vi "WSVCAP SHL Host LL I2C Write.vi"(0 "C1 Data Out [DUT Ordered]":u8[][](array[numeric]) format="%.0x", 1 "Wait Ticks":u32, 2 "Slave Address":u8, 3 "Socket Mask [U64]":u64=1 format="%06x", 11 "error in":errorcluster, 12 "Sub Address":u8=20, 13 "UUT Set (0/1)":u8, 14 "FPGA":T1) -> (10 "Status":u8[](array[numeric]), 15 "error out":errorcluster)   [LabVIEW 2017]
uses:
  Type Defs/WSVCAP SHL FPGA Enum.ctl
  Type Defs/WSVCAP SHL Top Level Write Read State Enum.ctl
  Type Defs/WSVCAP SHL Transaction Enum.ctl
  Type Defs/WSVCAP SHL Top Level Control Enum.ctl
  Type Defs/WSVCAP SHL State.ctl
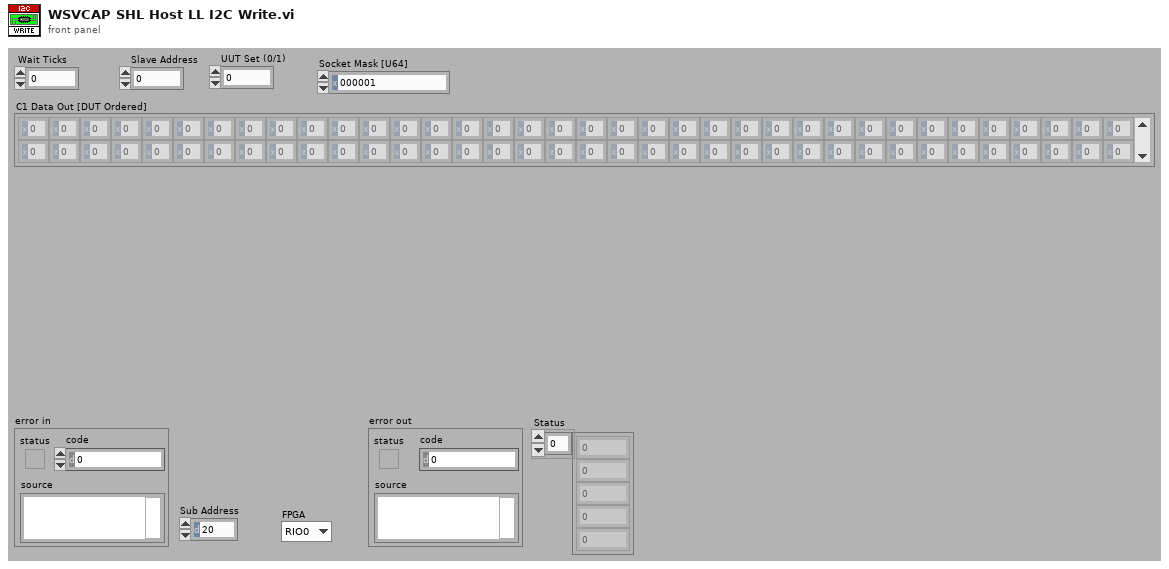
[diagram p1: front panel]
types:
  T1 = typedef "WSVCAP SHL FPGA Enum.ctl" = enum16{"RIO0", "RIO1"}
  T2 = typedef "WSVCAP SHL Top Level Write Read State Enum.ctl" = enum16{"Start", "Write", "Read", "Get Status", "Wait Until Done"}
  T3 = typedef "WSVCAP SHL Top Level Control Enum.ctl" = enum16{"Start", "Cmd", "Transaction", "Wait Ticks", "Socket Mask", "UUT Set", "Slave Address", "Sub Address", "Bytes to Write", "Bytes to Read", "Write Data", "Write Flag", "Read Data", "Read Flag", "Ack Read", "Read Status Flag", "Ack Read Status", "Status", "Cycle Count", "Stop Cycle", "Exit"}
  T4 = typedef "WSVCAP SHL Transaction Enum.ctl" = enum16{"I2C-Read Data", "I2C-Write Data", "RFFE-Ext Write", "RFFE-Ext Read", "SRL-Write Data"}
  T5 = typedef "WSVCAP SHL State.ctl" = enum8{"Idle", "Transfer Data"}
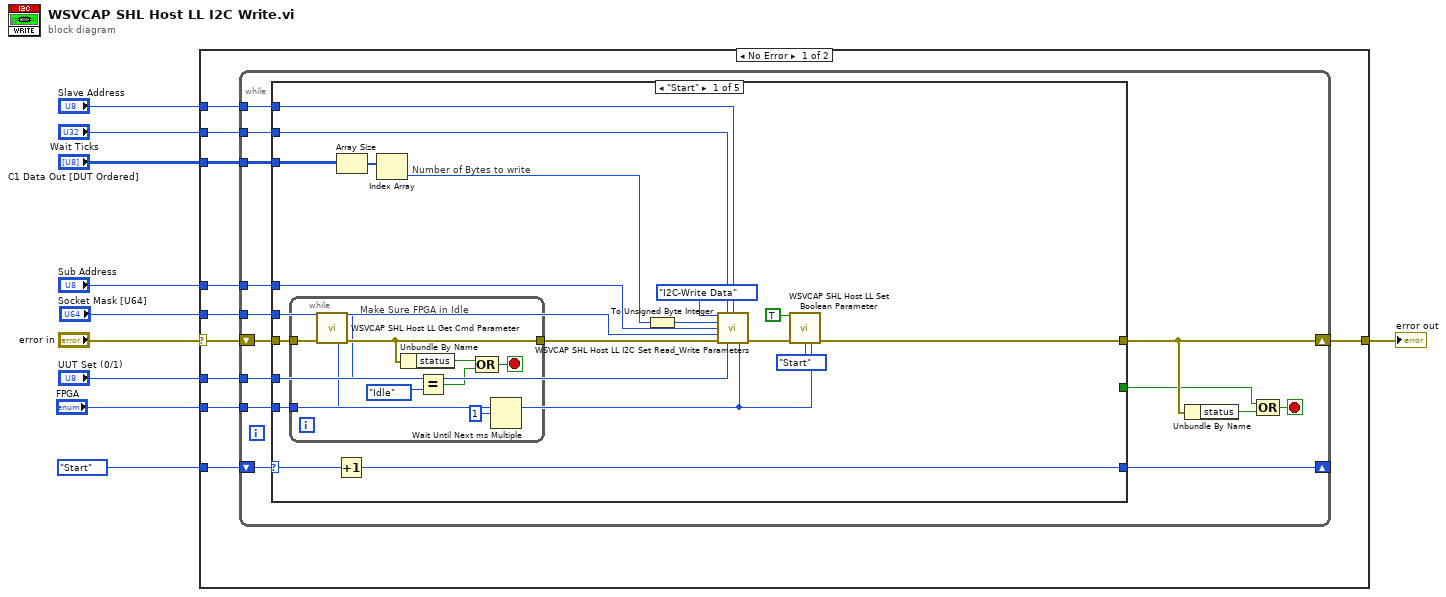
[diagram p0: block diagram]
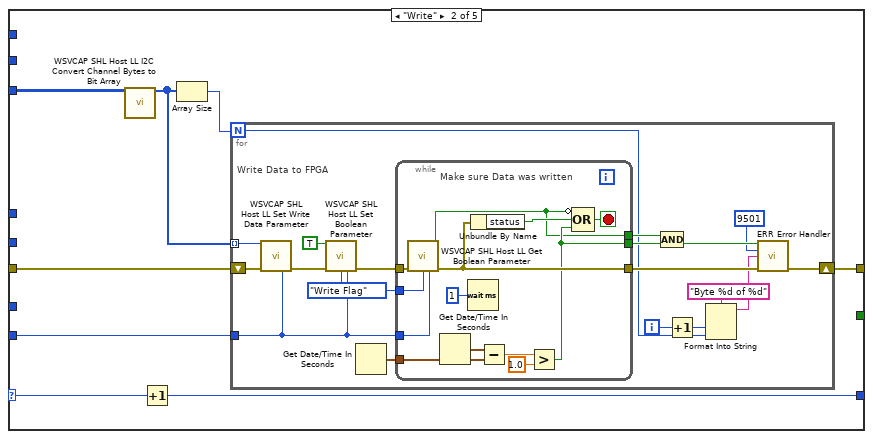
[diagram p2: hidden frame]
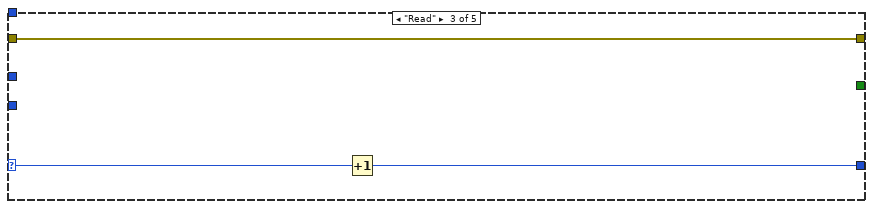
[diagram p3: hidden frame]
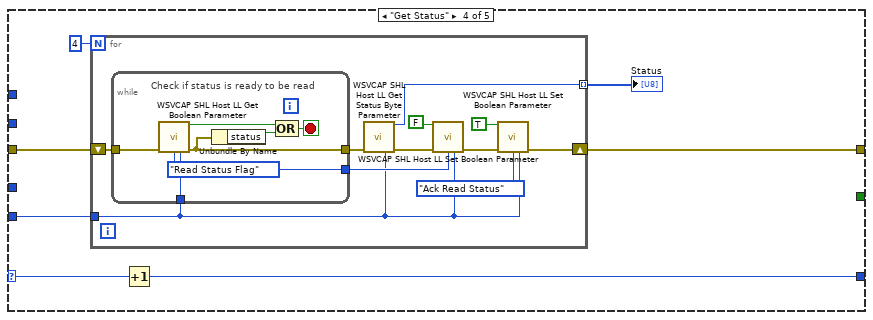
[diagram p4: hidden frame]
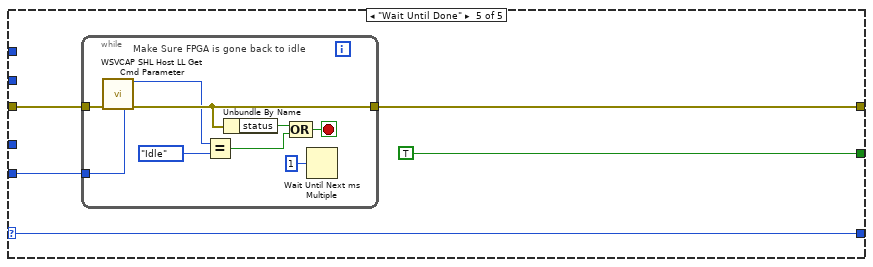
[diagram p5: hidden frame]
diagram:
  n1 = case shown="No Error" "error in" {
    selector: "error in" -> [w15 w144]
    tunnel: [w20 w144] -> w10
    tunnel: WSVCAP_SHL_Top_Level_Write_Read_State_Enum."Start" ("Write Read State") -> [w19 _]
    tunnel: "C1 Data Out [DUT Ordered]" -> [w18 _]
    tunnel: "Sub Address" -> [w17 _]
    tunnel: "Socket Mask [U64]" -> [w16 _]
    tunnel: "Wait Ticks" -> [w14 _]
    tunnel: "Slave Address" -> [w13 _]
    tunnel: "UUT Set (0/1)" -> [w12 _]
    tunnel: "FPGA" -> [w11 _]
    frame No Error {
      n2 = while {
        shift-right: [w33] -> w20
        shift-left: w15 -> [w34]
        shift-right: [w28] -> _
        shift-left: w19 -> [w29]
        tunnel: w18 -> [w27]
        tunnel: w17 -> [w26]
        tunnel: w16 -> [w25]
        tunnel: w14 -> [w24]
        tunnel: w13 -> [w23]
        tunnel: w12 -> [w22]
        tunnel: w11 -> [w21]
        stop <- w30 stop-if-true
        n3 = case shown="\"Start\"" w29 {
          selector: w29 -> [w51 w67 w103 w109 w132]
          tunnel: w34 -> [w52 w64 w104 w111 w134]
          tunnel: [w48 w69 w104 w110 w133] -> w33
          tunnel: [_ _ _ _ TRUE] -> w32
          tunnel: [w50 w68 w102 w108 w132] -> w28
          tunnel: w27 -> [w44 w63 _ _ _]
          tunnel: w26 -> [w40 _ _ _ _]
          tunnel: w25 -> [w39 _ _ _ _]
          tunnel: w24 -> [w38 _ _ _ _]
          tunnel: w23 -> [w37 _ _ _ _]
          tunnel: w22 -> [w36 _ _ _ _]
          tunnel: w21 -> [w35 w62 _ w105 w130]
          frame "Start" {
            # "Number of Bytes to write"
            n4 = while {
              tunnel: w52 -> [w57]
              tunnel: [w56] -> w49
              tunnel: w35 -> [w53]
              stop <- w61 stop-if-true
              # "Make Sure FPGA in Idle"
              n5 = call "WSVCAP SHL Host LL Get Cmd Parameter.vi"("error in (no error)"=w57, "FPGA"=w53) -> ("I2C_Cmd"=w55:T5, "error out"=w56:errorcluster)  [unwired: 12 in]
              n6 = Unbundle By Name(w56) -> ("status"=w54:bool)
              n7 = Equal?(x=w55, y=WSVCAP_SHL_State."Idle" ("Type")) -> (x = y?=w59:bool)
              n8 = Compound Arithmetic op=OR(w54, w59) -> (w61:bool)
              n9 = Wait Until Next ms Multiple(millisecond multiple=u32 1) -> ()  [unwired: 1 out]
            }
            n10 = Increment(x=w51) -> (x+1=w50:T2)
            n11 = Array Size(array=w44) -> (size(s)=w43:i32[])
            n12 = Index Array(array=w43) -> (element=w42:i32)  [unwired: 1 in]
            n13 = To Unsigned Byte Integer(number=w42) -> (unsigned 8bit integer=w41:u8)
            n14 = call "WSVCAP SHL Host LL I2C Set Read_Write Parameters.vi"("Transaction"=WSVCAP_SHL_Transaction_Enum."I2C-Write Data", "Wait Ticks"=w38, "Slave Address"=w37, "Bytes"=w41, "Sub Address [U8]"=w40, "Socket Mask [U64]"=w39, "error in (no error)"=w49, "UUT Set (0/1)"=w36, "FPGA"=w35) -> ("error out"=w48:errorcluster)  [unwired: 6 in]
            n15 = call "WSVCAP SHL Host LL Set Boolean Parameter.vi"("Boolean In"=TRUE, "error in (no error)"=w48, "FPGA Top Level Control"=WSVCAP_SHL_Top_Level_Control_Enum."Start", "FPGA"=w35) -> ()  [unwired: 11 in, 1 out]
          }
          frame "Write" {
            # "Write Data to FPGA"
            n16 = call "WSVCAP SHL Host LL I2C Convert Channel Bytes to Bit Array.vi"("C1 Data Out"=w63) -> ("Write Data"=w65:u64[])  [unwired: 14 in]
            n17 = Increment(x=w67) -> (x+1=w68:T2)
            n18 = Array Size(array=w65) -> (size(s)=w66:i32)
            n19 = for {
              N: w66 -> [w72]
              shift-right: [w80] -> w69
              shift-left: w64 -> [w88]
              tunnel: w65 -> [w87] mode=indexing
              tunnel: w62 -> [w70]
              i -> [w75]
              w83 = WSVCAP_SHL_Top_Level_Control_Enum."Write Flag" ("FPGA Top Level Control")
              n20 = call "WSVCAP SHL Host LL Set Write Data Parameter.vi"("Write Byte In"=w87, "error in (no error)"=w88, "FPGA"=w70) -> ("error out"=w86:errorcluster)  [unwired: 12 in]
              n21 = call "WSVCAP SHL Host LL Set Boolean Parameter.vi"("Boolean In"=TRUE, "error in (no error)"=w86, "FPGA Top Level Control"=w83, "FPGA"=w70) -> ("error out"=w84:errorcluster)  [unwired: 11 in]
              n22 = Get Date/Time In Seconds() -> (seconds since 1Jan1904=w82:timestamp)
              n23 = while {
                tunnel: w84 -> [w99]
                tunnel: [w98] -> w81
                tunnel: w83 -> [w97]
                tunnel: w82 -> [w94]
                tunnel: [w91] -> w79
                tunnel: [w90] -> w78
                tunnel: w70 -> [w89]
                stop <- w101 stop-if-true
                # "Make sure Data was written"
                n24 = call "WSVCAP SHL Host LL Get Boolean Parameter.vi"("error in (no error)"=w99, "FPGA Top Level Control"=w97, "FPGA"=w89) -> ("Boolean Out"=w90:bool, "error out"=w98:errorcluster)  [unwired: 11 in]
                n25 = Get Date/Time In Seconds() -> (seconds since 1Jan1904=w95:timestamp)
                n26 = Wait (ms)(milliseconds to wait=u32 1) -> ()  [unwired: 1 out]
                n27 = Unbundle By Name(w98) -> ("status"=w96:bool)
                n28 = Subtract(x=w95, y=w94) -> (x-y=w93:dbl)
                n29 = Greater?(x=w93, y=1.0) -> (0:w91:bool)
                n30 = Compound Arithmetic op=OR(invert w90, w96, w91) -> (w101:bool)
              }
              n31 = Compound Arithmetic op=AND(w78, w79) -> (w77:bool)
              n32 = Increment(x=w75) -> (x+1=w71:i32)
              n33 = Format Into String(format string="Byte %d of %d", w71, w72) -> (resulting string=w74:string)  [unwired: 2 in, 1 out]
              n34 = call "ERR Error Handler.vi"("Error Status"=w77, "Error Code"=9501, "Cause Of Error"=w74, "Error In (no error)"=w81) -> ("Error Out"=w80:errorcluster)  [unwired: 11 in]
            }
          }
          frame "Read" {
            n35 = Increment(x=w103) -> (x+1=w102:T2)
          }
          frame "Get Status" {
            n36 = for {
              N: 4 -> [_]
              shift-right: [w121] -> w110
              shift-left: w111 -> [w122]
              tunnel: [w113] -> w106 mode=indexing
              tunnel: w105 -> [w112]
              n37 = while {
                tunnel: w122 -> [w127]
                tunnel: [w126] -> w120
                tunnel: [w124] -> w118
                tunnel: w112 -> [w123]
                stop <- w129 stop-if-true
                w124 = WSVCAP_SHL_Top_Level_Control_Enum."Read Status Flag" ("FPGA Top Level Control")
                # "Check if status is ready to be read"
                n38 = call "WSVCAP SHL Host LL Get Boolean Parameter.vi"("error in (no error)"=w127, "FPGA Top Level Control"=w124, "FPGA"=w123) -> ("Boolean Out"=w128:bool, "error out"=w126:errorcluster)  [unwired: 11 in]
                n39 = Unbundle By Name(w126) -> ("status"=w125:bool)
                n40 = Compound Arithmetic op=OR(w128, w125) -> (w129:bool)
              }
              n41 = call "WSVCAP SHL Host LL Get Status Byte Parameter.vi"("error in (no error)"=w120, "FPGA"=w112) -> ("I2C Status Byte"=w113:u8, "error out"=w119:errorcluster)  [unwired: 12 in]
              n42 = call "WSVCAP SHL Host LL Set Boolean Parameter.vi"("Boolean In"=FALSE ("Read Flag"), "error in (no error)"=w119, "FPGA Top Level Control"=w118, "FPGA"=w112) -> ("error out"=w114:errorcluster)  [unwired: 11 in]
              n43 = call "WSVCAP SHL Host LL Set Boolean Parameter.vi"("Boolean In"=TRUE ("Write Flag"), "error in (no error)"=w114, "FPGA Top Level Control"=WSVCAP_SHL_Top_Level_Control_Enum."Ack Read Status", "FPGA"=w112) -> ("error out"=w121:errorcluster)  [unwired: 11 in]
            }
            "Status" <- w106
            n44 = Increment(x=w109) -> (x+1=w108:T2)
          }
          frame "Wait Until Done" {
            n45 = while {
              tunnel: w134 -> [w138]
              tunnel: [w137] -> w133
              tunnel: w130 -> [w135]
              stop <- w140 stop-if-true
              # "Make Sure FPGA is gone back to idle"
              n46 = call "WSVCAP SHL Host LL Get Cmd Parameter.vi"("error in (no error)"=w138, "FPGA"=w135) -> ("I2C_Cmd"=w136:T5, "error out"=w137:errorcluster)  [unwired: 12 in]
              n47 = Equal?(x=w136, y=WSVCAP_SHL_State."Idle") -> (x = y?=w141:bool)
              n48 = Unbundle By Name(w137) -> ("status"=w142:bool)
              n49 = Compound Arithmetic op=OR(w142, w141) -> (w140:bool)
              n50 = Wait Until Next ms Multiple(millisecond multiple=u32 1) -> ()  [unwired: 1 out]
            }
          }
        }
        n51 = Unbundle By Name(w33) -> ("status"=w31:bool)
        n52 = Compound Arithmetic op=OR(w32, w31) -> (w30:bool)
      }
    }
    frame Error {
    }
  }
  "error out" <- w10
